vi "SetColorMode.vi"(6 "Name":refnum<vi>, 9 "Bayer pattern":refnum<vi>, 10 "Color (Off/On)":refnum<vi>, 11 ".NET Refnum in":refnum<k24>) -> ()   [LabVIEW 2018]
uses:
  D:/SVN/PM/sdk/AppSamples/LabVIEWSamples/trunk/Release/2018/Dependencies/PVCamNET.dll
  Dependencies/PVCamNET.dll
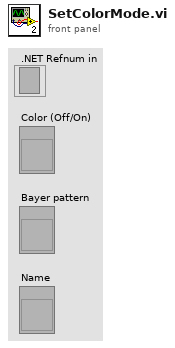
[diagram p1: front panel]
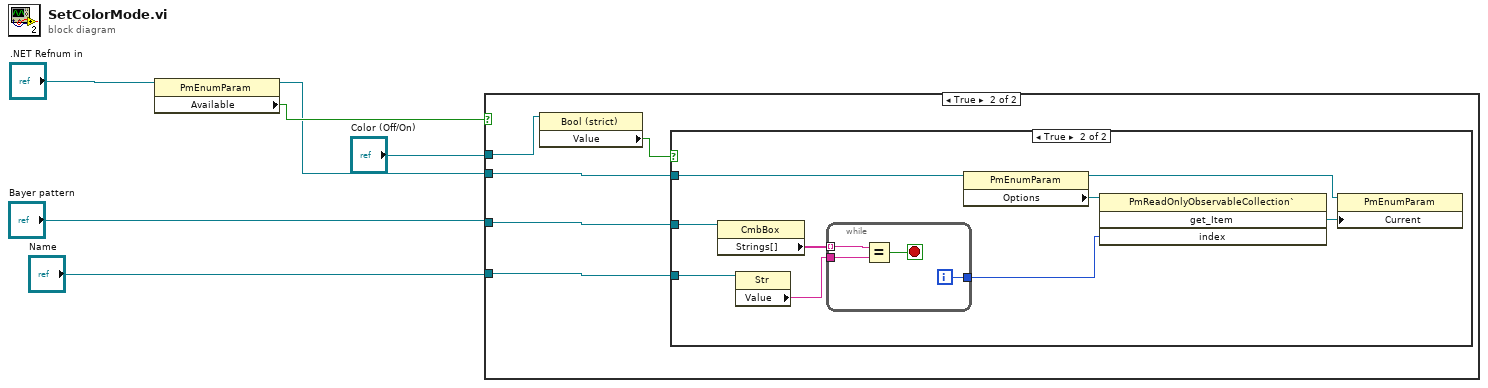
[diagram p0: block diagram]
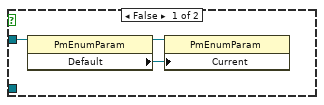
[diagram p3: hidden frame]
diagram:
  n1 = property class="PmEnumParam"(reference=".NET Refnum in") -> (reference out=w3:refnum<k24>, "Available"=w4:bool)  [unwired: 1 in, 1 out]
  n2 = case shown="True" w4 {
    tunnel: w3 -> [_ w11]
    tunnel: "Bayer pattern" -> [_ w10]
    tunnel: "Color (Off/On)" -> [_ w7]
    tunnel: "Name" -> [_ w9]
    frame False {
    }
    frame True {
      n3 = property class="Bool (strict)"(reference=w7) -> ("Value"=w8:bool)  [unwired: 1 in, 2 out]
      n4 = case shown="True" w8 {
        tunnel: w11 -> [w14 w22]
        tunnel: w10 -> [_ w17]
        tunnel: w9 -> [_ w16]
        frame False {
          n5 = property class="PmEnumParam"(reference=w14) -> (reference out=w12:refnum<k24>, "Default"=w13:refnum<k24>)  [unwired: 1 in, 1 out]
          n6 = property class="PmEnumParam"(reference=w12, "Current"=w13) -> ()  [unwired: 1 in, 2 out]
        }
        frame True {
          n7 = property class="CmbBox"(reference=w17) -> ("Strings[]"=w23:string[])  [unwired: 1 in, 2 out]
          n8 = property class="Str"(reference=w16) -> ("Value"=w15:string)  [unwired: 1 in, 2 out]
          n9 = while {
            tunnel: w23 -> [w27] mode=indexing
            tunnel: [w25] -> w20
            tunnel: w15 -> [w24]
            i -> [w25]
            stop <- w26 stop-if-true
            n10 = Equal?(x=w27, y=w24) -> (x = y?=w26:bool)
          }
          n11 = property class="PmEnumParam"(reference=w22) -> (reference out=w18:refnum<k24>, "Options"=w21:refnum<k24>)  [unwired: 1 in, 1 out]
          n12 = invoke class="PmReadOnlyObservableCollection`" method="get_Item"(reference=w21, "index"=w20) -> ("get_Item"=w19:refnum<k24>)  [unwired: 2 in, 3 out]
          n13 = property class="PmEnumParam"(reference=w18, "Current"=w19) -> ()  [unwired: 1 in, 2 out]
        }
      }
    }
  }
